vi "Unflatten Message Class.vi"(7 "Message Type":refnum<class "Message.lvclass">, 8 "error in (no error)":errorcluster, 9 "Data":variant, 11 "Module in":refnum<class "Module.lvclass">) -> (0 "error out":errorcluster, 2 "Message":refnum<class "Message.lvclass">, 3 "Module out":refnum<class "Module.lvclass">, 5 "TcpPayload":T1)   [LabVIEW 2020, in "Volatus.lvlib" / "Module.lvclass"]
uses:
  Module.lvclass
  Module.lvclass/Module.ctl
  lv-vecto/Vecto/proto/TcpPayload/Data.ctl
  lv-vecto/Vecto/proto/TcpPayload/TcpPayload.lvlib
  lv-protoc/LV-Proto/Message/Message.lvclass
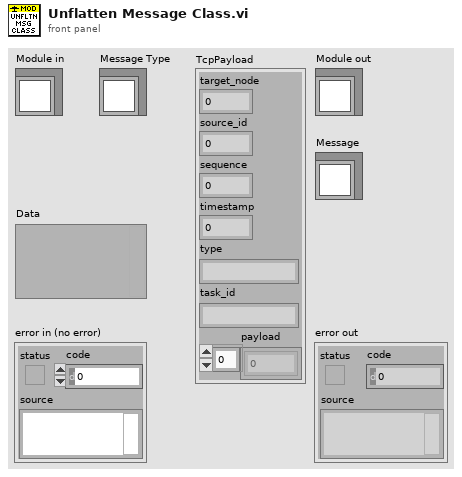
[diagram p1: front panel]
types:
  T1 = typedef "TcpPayload.lvlib/Data.ctl" = cluster{"target_node":u32, "source_id":u32, "sequence":u32, "timestamp":u64, "type":string, "task_id":string, "payload":u8[]}
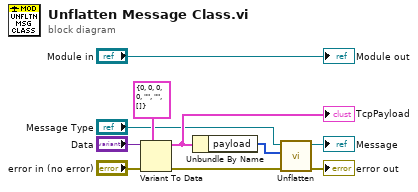
[diagram p0: block diagram]
diagram:
  n1 = Variant To Data(error in="error in (no error)", type=T1 {"target_node"=0, "source_id"=0, "sequence"=0, "timestamp"=0, "type"="", "task_id"="", "payload"=[]} ("TcpPayload"), Variant="Data") -> (data=w6:T1, error out=w4:errorcluster)
  "TcpPayload" <- w6
  n2 = Unbundle By Name(w6) -> ("payload"=w5:u8[])
  n3 = call-dynamic "Unflatten.vi"("error in (no error)"=w4, "Buffer"=w5, "Message in"="Message Type") -> ("error out"=→"error out":errorcluster, "Message out"=→"Message":refnum<class "Message.lvclass">)  [unwired: 7 in]
  "Module out" <- "Module in"
